vi "Main.vi"() -> ()   [LabVIEW 2019]
uses:
  Sub VIs/State Estimator/Measurements.ctl
  Sub VIs/IMU/IMU Data.ctl
  Sub VIs/Steering Motor Encoder/Steering Motor Encoder Data.ctl
  Sub VIs/GNSS/GNSS Data.ctl
  Sub VIs/State Estimator/State Estimate.ctl
  Sub VIs/Logging/Log Level.ctl
  <vilib>/Platform/TimedLoop/XDataNode/timing_clust.ctl
  <vilib>/Platform/TimedLoop/XDataNode/nitl_modes.ctl
  <vilib>/Platform/TimedLoop/XDataNode/wakeup.ctl
  <vilib>/platform/TimedLoop/XDataNode/XDataNode.xnode
  <vilib>/Platform/TimedLoop/XDataNode/XDNodeRunTimeDep.lvlib
panel:
  in  "Enable Steering Motor":bool
  out "Steering Motor Enabled":bool
  out "State Estimate (Debug)":T1
  out "Measurements (Debug)":T2
  out "Abort":bool
  in  "Reset Counter":bool
  in  "Stop Button":bool
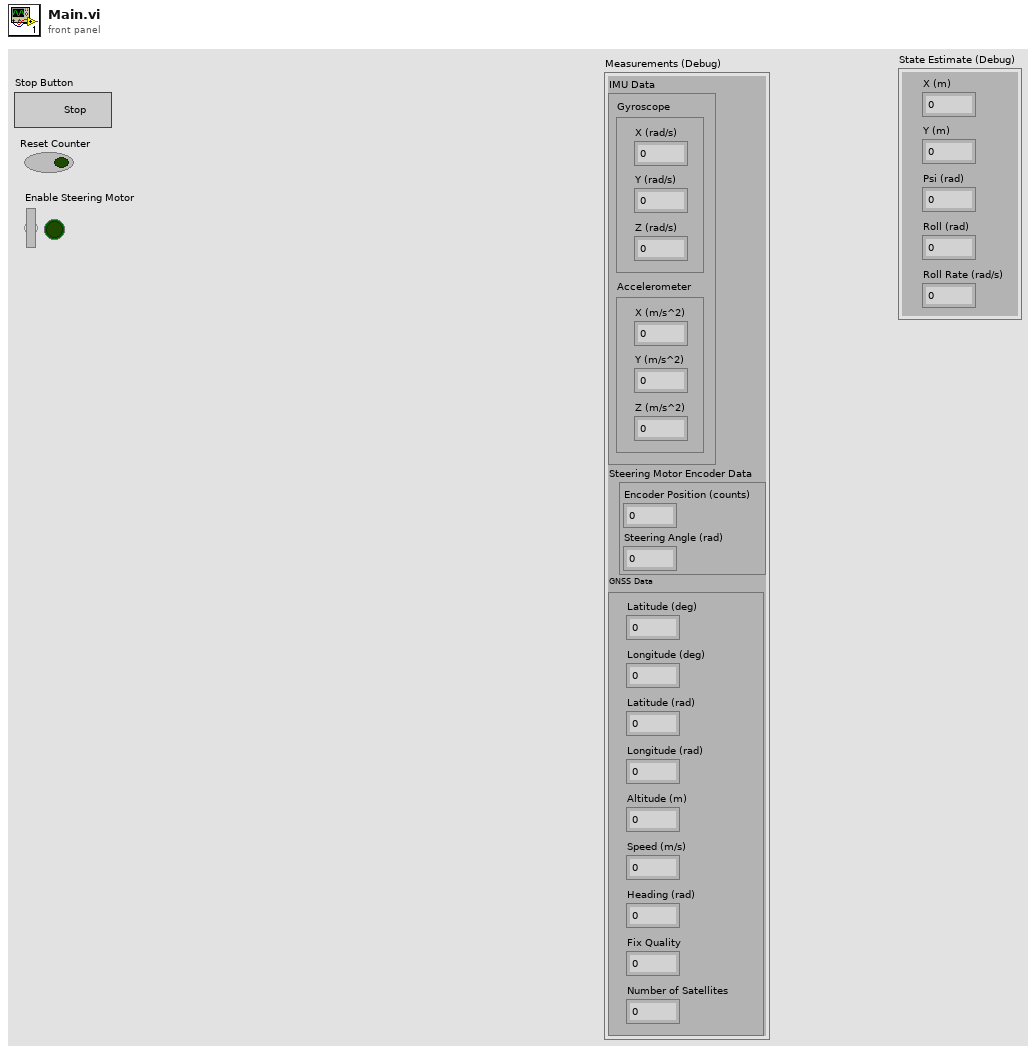
[diagram p1: front panel]
types:
  T1 = typedef "State Estimate.ctl" = cluster{"X (m)":dbl, "Y (m)":dbl, "Psi (rad)":dbl, "Roll (rad)":dbl, "Roll Rate (rad/s)":dbl}
  T2 = typedef "Measurements.ctl" = cluster{"IMU Data":T3, "Steering Motor Encoder Data":T4, "GNSS Data":T5}
  T3 = typedef "IMU Data.ctl" = cluster{"Gyroscope":cluster{"X (rad/s)":dbl, "Y (rad/s)":dbl, "Z (rad/s)":dbl}, "Accelerometer":cluster{"X (m/s^2)":dbl, "Y (m/s^2)":dbl, "Z (m/s^2)":dbl}}
  T4 = typedef "Steering Motor Encoder Data.ctl" = cluster{"Encoder Position (counts)":i32, "Steering Angle (rad)":dbl}
  T5 = typedef "GNSS Data.ctl" = cluster{"Latitude (rad)":dbl, "Longitude (rad)":dbl, "Altitude (m)":dbl, "Speed (m/s)":dbl, "Heading (rad)":dbl, "Fix Quality":i32, "Number of Satellites":i32, "Latitude (deg)":dbl, "Longitude (deg)":dbl}
  T6 = typedef "XDNodeRunTimeDep.lvlib/timing_clust.ctl" = cluster{"Expected End [f-1]":u64, "Actual End [f-1]":u64, "Finished Late? [f-1]":bool, "Expected End [i-1]":u64, "Actual End [i-1]":u64, "Finished Late? [i-1]":bool, "Expected Start [i]":u64, "Actual Start [i]":u64, "Expected Start [f]":u64, "Actual Start [f]":u64, "Source Name":string, "Structure Name":string, "Period":i64, "Deadline":i64, "Offset":i64, "Start":i64, "Priority":i32, "Timeout":i32, "Mode":T7, "Wakeup Reason":T8, "Error":errorcluster, "Source Type":string, "Secondary Source Type":string, "Global End Time":u64, "Global Start Time":u64, "Frame Duration":u64, "Iteration Duration":u64, "Assigned CPU":i32, "I/O Scan Engine Mode":u32}
  T7 = typedef "XDNodeRunTimeDep.lvlib/nitl_modes.ctl" = enum32{"No Change", "Process missed periods, maintain original phase", "Discard missed periods, maintain original phase", "Process missed periods, ignore original phase", "Discard missed periods, ignore original phase"}
  T8 = typedef "XDNodeRunTimeDep.lvlib/wakeup.ctl" = enum32{"Normal", "Aborted", "Asynchronous wakeup", "Timing source error", "Timed loop error", "Timeout"}
  T9 = typedef "Log Level.ctl" = enum16{"Error", "Warning", "Info"}
  T10 = typedef "Configuration.ctl" = cluster{"Accelerometer Bias":cluster{"X (m/s)":dbl, "Y (m/s)":dbl, "Z (m/s)":dbl}, "Gyroscope Bias":cluster{"X (m/s)":dbl, "Y (m/s)":dbl, "Z (m/s)":dbl}, "Steering Motor Gear Ratio":dbl, "Steering Pully Gear Ratio":dbl, "Steering Encoder CPR":dbl, "Steering Motor Max RPM":dbl, "Wheelbase (m)":dbl, "Fork Angle (rad)":dbl, "Balancing Controller":cluster{"Kp (/s)":dbl, "Kd (1)":dbl}, "Max Allowed Steering Angle (rad)":dbl, "Task Periods":cluster{"Emergency Stop (us)":i64, "IMU (us)":i64, "Steering Motor Encoder (us)":i64, "State Estimator (us)":i64, "Balancing Controller (us)":i64, "GNSS (us)":i64, "Logging (us)":i64}}
  T11 = typedef "IMU Handle.ctl" = cluster{"I2C address":u8}
  T12 = typedef "GNSS Handle.ctl" = cluster{"VISA Resource Name":refnum<visa-resource-name>}
  T13 = typedef "Steering Motor Handle.ctl" = cluster{"Dummy":dbl}
  T14 = typedef "Log Handle.ctl" = cluster{"Data File":refnum<file>, "Event File":refnum<file>}
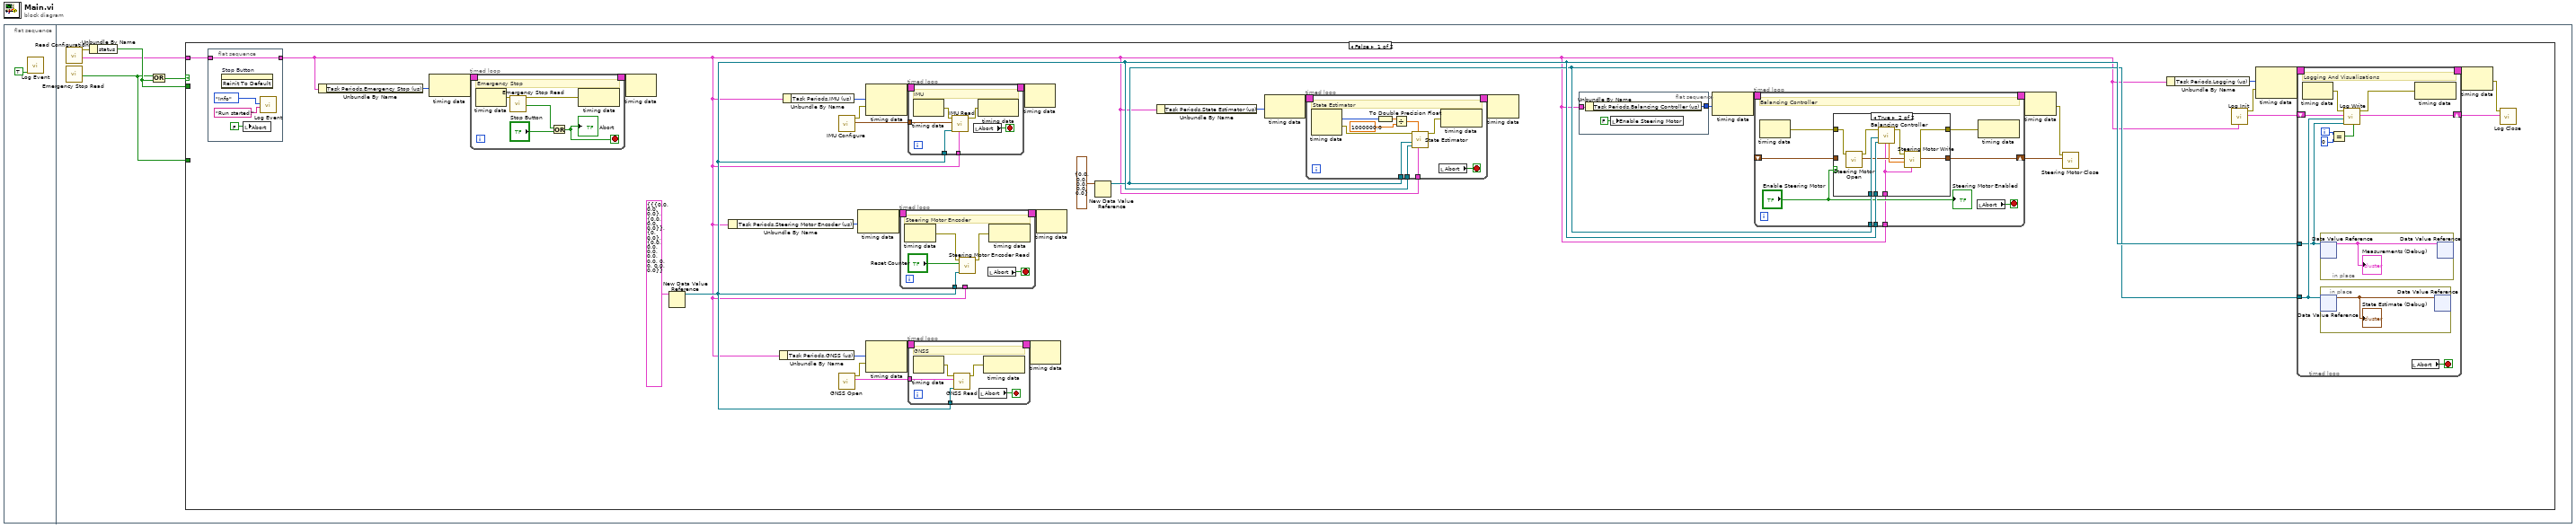
[diagram p0: block diagram]
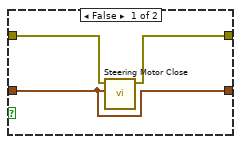
[diagram p2: hidden frame]
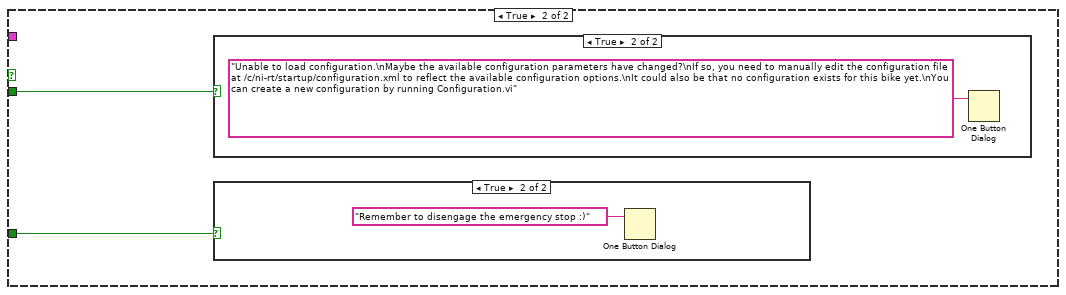
[diagram p3: hidden frame]
diagram:
  n1 = flat-sequence {
    frame #0 {
      n2 = call "Log Event.vi"("Clear Log"=TRUE) -> ()  [unwired: 10 in, 1 out]
    }
    frame #1 {
      n3 = call "Read Configuration.vi"() -> ("Configuration"=w3:T10, "Error Out"=w2:errorcluster)  [unwired: 10 in]
      n4 = call "Emergency Stop Read.vi"() -> ("Emergency Stop"=w4:bool)  [unwired: 10 in, 1 out]
      n5 = Unbundle By Name(w2) -> ("status"=w5:bool)
      n6 = Compound Arithmetic op=OR(w4, w5) -> (w6:bool)
      n7 = case shown="False" w6 {
        tunnel: w5 -> [_ w185]
        tunnel: w4 -> [_ w186]
        tunnel: w3 -> [w15 _]
        frame False {
          n8 = flat-sequence {
            tunnel: [w181] -> w7
            tunnel: w15 -> [w181]
            frame #0 {
              n9 = invoke on="Stop Button" class="Bool (strict)" method="Reinit To Default"() -> ()  [unwired: 3 in, 3 out]
              n10 = local write "Abort"(FALSE ("Abort")) -> ()
              n11 = call "Log Event.vi"("Message"="Run started!", "Log Level"=Log_Level."Info") -> ()  [unwired: 9 in, 1 out]
            }
          }
          n12 = Unbundle By Name(w7) -> ("Task Periods.Emergency Stop (us)"=w39:i64)
          n13 = node-c288(w39) -> (w38:T6)
          n14 = timed-loop {
            timing: w38 -> [_]
            timing-out: [_] -> w37
            stop <- w167 stop-if-true
            # "Emergency Stop"
            n15 = node-c288() -> (w171:errorcluster)  [unwired: 1 in]
            n16 = call "Emergency Stop Read.vi"("Error In"=w171) -> ("Emergency Stop"=w169:bool, "Error Out"=w170:errorcluster)  [unwired: 9 in]
            n17 = Or(x=w169, y="Stop Button") -> (x .or. y?=w167:bool)
            "Abort" <- w167
            n18 = node-c288(w170) -> ()  [unwired: 1 out]
          }
          n19 = node-c288(w37) -> ()  [unwired: 1 out]
          n20 = New Data Value Reference(data value=T2 {"IMU Data"={"Gyroscope"={"X (rad/s)"=0.0, "Y (rad/s)"=0.0, "Z (rad/s)"=0.0}, "Accelerometer"={"X (m/s^2)"=0.0, "Y (m/s^2)"=0.0, "Z (m/s^2)"=0.0}}, "Steering Motor Encoder Data"={"Encoder Position (counts)"=0, "Steering Angle (rad)"=0.0}, "GNSS Data"={"Latitude (rad)"=0.0, "Longitude (rad)"=0.0, "Altitude (m)"=0.0, "Speed (m/s)"=0.0, "Heading (rad)"=0.0, "Fix Quality"=0, "Number of Satellites"=0, "Latitude (deg)"=0.0, "Longitude (deg)"=0.0}} ("Cluster")) -> (data value reference=w41:refnum<data-value>)  [unwired: 1 in, 1 out]
          n21 = Unbundle By Name(w7) -> ("Task Periods.Steering Motor Encoder (us)"=w23:i64)
          n22 = Unbundle By Name(w7) -> ("Task Periods.GNSS (us)"=w20:i64)
          n23 = Unbundle By Name(w7) -> ("Task Periods.IMU (us)"=w24:i64)
          n24 = call "IMU Configure.vi"() -> ("IMU Handle"=w25:T11, "Error Out"=w26:errorcluster)  [unwired: 10 in]
          n25 = call "GNSS Open.vi"() -> ("GNSS Handle"=w21:T12, "Error Out"=w22:errorcluster)  [unwired: 10 in]
          n26 = node-c288(w23) -> (w30:T6)
          n27 = node-c288(w24, w26) -> (w32:T6)
          n28 = node-c288(w20, w22) -> (w28:T6)
          n29 = timed-loop {
            timing: w30 -> [_]
            timing-out: [_] -> w29
            tunnel: w41 -> [w102]
            tunnel: w7 -> [_]
            stop <- w103 stop-if-true
            # "Steering Motor Encoder"
            n30 = node-c288() -> (w106:errorcluster)  [unwired: 1 in]
            n31 = call "Steering Motor Encoder Read.vi"("Measurement In"=w102, "Reset Counter"="Reset Counter", "Error In"=w106) -> ("Error Out"=w105:errorcluster)  [unwired: 6 in, 2 out]
            n32 = local read "Abort"() -> (w103:bool)
            n33 = node-c288(w105) -> ()  [unwired: 1 out]
          }
          n34 = timed-loop {
            timing: w32 -> [_]
            timing-out: [_] -> w31
            tunnel: w25 -> [w119]
            tunnel: w41 -> [w117]
            tunnel: w7 -> [w116]
            stop <- w118 stop-if-true
            # "IMU"
            n35 = node-c288() -> (w121:errorcluster)  [unwired: 1 in]
            n36 = call "IMU Read.vi"("Configuration"=w116, "Measurement In"=w117, "IMU Handle"=w119, "Error In"=w121) -> ("Error Out"=w120:errorcluster)  [unwired: 5 in, 2 out]
            n37 = local read "Abort"() -> (w118:bool)
            n38 = node-c288(w120) -> ()  [unwired: 1 out]
          }
          n39 = timed-loop {
            timing: w28 -> [_]
            timing-out: [_] -> w27
            tunnel: w21 -> [w91]
            tunnel: w41 -> [w87]
            stop <- w88 stop-if-true
            # "GNSS"
            n40 = node-c288() -> (w90:errorcluster)  [unwired: 1 in]
            n41 = call "GNSS Read.vi"("Measurement In"=w87, "GNSS Handle"=w91, "Error In"=w90) -> ("Error Out"=w89:errorcluster)  [unwired: 6 in, 2 out]
            n42 = local read "Abort"() -> (w88:bool)
            n43 = node-c288(w89) -> ()  [unwired: 1 out]
          }
          n44 = node-c288(w31) -> ()  [unwired: 1 out]
          n45 = node-c288(w27) -> ()  [unwired: 1 out]
          n46 = node-c288(w29) -> ()  [unwired: 1 out]
          n47 = New Data Value Reference(data value=T1 {"X (m)"=0.0, "Y (m)"=0.0, "Psi (rad)"=0.0, "Roll (rad)"=0.0, "Roll Rate (rad/s)"=0.0} ("State Estimate")) -> (data value reference=w40:refnum<data-value>)  [unwired: 1 in, 1 out]
          n48 = Unbundle By Name(w7) -> ("Task Periods.State Estimator (us)"=w17:i64)
          n49 = node-c288(w17) -> (w19:T6)
          n50 = timed-loop {
            timing: w19 -> [_]
            timing-out: [_] -> w18
            tunnel: w41 -> [w69]
            tunnel: w40 -> [w68]
            tunnel: w7 -> [w67]
            stop <- w76 stop-if-true
            # "State Estimator"
            n51 = node-c288() -> (w73:i64, w75:errorcluster)  [unwired: 1 in]
            n52 = To Double Precision Float(number=w73) -> (double precision float=w72:dbl)
            n53 = Divide(x=w72, y=1000000.0) -> (x/y=w70:dbl)
            n54 = call "State Estimator.vi"("Configuration"=w67, "Ts"=w70, "Measurement In"=w69, "State Estimate In"=w68, "Error In"=w75) -> ("Error out"=w74:errorcluster)  [unwired: 4 in, 2 out]
            n55 = local read "Abort"() -> (w76:bool)
            n56 = node-c288(w74) -> ()  [unwired: 1 out]
          }
          n57 = node-c288(w18) -> ()  [unwired: 1 out]
          n58 = flat-sequence {
            tunnel: [w133] -> w16
            tunnel: w7 -> [w132]
            frame #0 {
              n59 = Unbundle By Name(w132) -> ("Task Periods.Balancing Controller (us)"=w133:i64)
              n60 = local write "Enable Steering Motor"(FALSE ("Enable Steering Motor")) -> ()
            }
          }
          n61 = node-c288(w16) -> (w36:T6)
          n62 = timed-loop {
            timing: w36 -> [_]
            timing-out: [_] -> w35
            tunnel: w40 -> [w139]
            tunnel: w41 -> [w138]
            shift-right: [w140] -> w34
            shift-left: _ -> [w136]
            tunnel: w7 -> [w135]
            stop <- w143 stop-if-true
            # "Balancing Controller"
            n63 = node-c288() -> (w142:errorcluster)  [unwired: 1 in]
            n64 = case shown="True" "Enable Steering Motor" {
              tunnel: w142 -> [w146 w150]
              tunnel: [w145 w155] -> w141
              tunnel: [w144 w154] -> w140
              tunnel: w139 -> [_ w152]
              tunnel: w138 -> [_ w151]
              tunnel: w136 -> [w144 _]
              tunnel: w135 -> [_ w147]
              frame False {
                n65 = call "Steering Motor Close.vi"("Steering Motor Handle"=w144, "Error In"=w146) -> ("Error Out"=w145:errorcluster)  [unwired: 9 in]
              }
              frame True {
                n66 = call "Steering Motor Open.vi"("Error In"=w150) -> ("Steering Motor Handle"=w148:T13, "Error Out"=w149:errorcluster)  [unwired: 9 in]
                n67 = call "Balancing Controller.vi"("Configuration"=w147, "Measurement In"=w151, "State Estimate In"=w152, "Error In"=w149) -> ("Error Out"=w156:errorcluster, "Steering Angle Rate (rad/s)"=w153:dbl)  [unwired: 4 in, 2 out]
                n68 = call "Steering Motor Write.vi"("Configuration"=w147, "Steering Bar Angular Velocity (rad/s)"=w153, "Steering Motor Handle In"=w148, "Error In"=w156) -> ("Steering Motor Handle Out"=w154:T13, "Error Out"=w155:errorcluster)  [unwired: 6 in]
              }
            }
            n69 = local read "Abort"() -> (w143:bool)
            n70 = node-c288(w141) -> ()  [unwired: 1 out]
            "Steering Motor Enabled" <- "Enable Steering Motor"
          }
          n71 = node-c288(w35) -> (w33:errorcluster)
          n72 = call "Steering Motor Close.vi"("Steering Motor Handle"=w34, "Error In"=w33) -> ()  [unwired: 9 in, 1 out]
          n73 = Unbundle By Name(w7) -> ("Task Periods.Logging (us)"=w12:i64)
          n74 = call "Log Init.vi"("Configuration"=w7) -> ("Log Handle"=w8:T14, "Error Out"=w11:errorcluster)  [unwired: 9 in]
          n75 = node-c288(w12, w11) -> (w14:T6)
          n76 = timed-loop {
            timing: w14 -> [_]
            timing-out: [_] -> w13
            tunnel: w41 -> [w48]
            tunnel: w40 -> [w49]
            shift-right: [w50] -> w9
            shift-left: w8 -> [w45]
            i -> [w47]
            stop <- w53 stop-if-true
            # "Logging And Visualisations"
            n77 = node-c288() -> (w52:errorcluster)  [unwired: 1 in]
            n78 = in-place {
              n79 = in-place-dvr #1(w48) -> (w55:T2)  [unwired: 1 out]
              "Measurements (Debug)" <- w55
              n80 = in-place-dvr #1(w55) -> ()  [unwired: 2 out]
            }
            n81 = in-place {
              n82 = in-place-dvr #2(w49) -> (w54:T1)  [unwired: 1 out]
              "State Estimate (Debug)" <- w54
              n83 = in-place-dvr #2(w54) -> ()  [unwired: 2 out]
            }
            n84 = Equal?(x=w47, y=0) -> (x = y?=w44:bool)
            n85 = call "Log Write.vi"("Write Header"=w44, "Measurement In"=w48, "State Estimate In"=w49, "Log Handle In"=w45, "Error In"=w52) -> ("Log Handle Out"=w50:T14, "Error Out"=w51:errorcluster)  [unwired: 2 in, 3 out]
            n86 = local read "Abort"() -> (w53:bool)
            n87 = node-c288(w51) -> ()  [unwired: 1 out]
          }
          n88 = node-c288(w13) -> (w10:errorcluster)
          n89 = call "Log Close.vi"("Log Handle In"=w9, "Error In"=w10) -> ()  [unwired: 9 in, 1 out]
        }
        frame True {
          n90 = case shown="True" w185 {
            frame False {
            }
            frame True {
              n91 = One Button Dialog(message="Unable to load configuration.\nMaybe the available configuration parameters have changed?\nIf so, you need to manually edit the configuration file at /c/ni-rt/startup/configuration.xml to reflect the available configuration options.\nIt could also be that no configuration exists for this bike yet.\nYou can create a new configuration by running Configuration.vi") -> ()  [unwired: 1 in, 1 out]
            }
          }
          n92 = case shown="True" w186 {
            frame False {
            }
            frame True {
              n93 = One Button Dialog(message="Remember to disengage the emergency stop :)") -> ()  [unwired: 1 in, 1 out]
            }
          }
        }
      }
    }
  }
